vi "Configure Trace Buffer.vi"(4 "Trace Buffer Size (100000)":i32=100000, 6 "Trace Time Rule (1: Absolute)":i32(ring)=1 items=["Delta", "Absolute"], 7 "Trace Buffer Control (1: Never)":i32(ring)=1 items=["Next", "Never"], 8 "error in (no error)":errorcluster, 9 "Trace Buffer Data (2: SENS)":i32(ring)=2 items=["MATH", "LIM", "SENS"], 10 "Channel (0: Channel 1)":i32(ring) items=["Channel 1", "Channel 2"], 11 "VISA resource name":refnum<visa-resource-name>) -> (0 "error out":errorcluster, 3 "VISA resource name out":refnum<visa-resource-name>)   [LabVIEW 2020, in "Agilent B2900 Series.lvlib"]
doc: "Configures the settings for Trace Buffer. \n\n<B>Note:</B>\nCommand \":TRAC[c]:FEED LIM\" is not applicable for Agilent models B2961A, B2962A, B2961B, B2962B, B2961C and B2962C."
uses:
  Agilent B2900 Series.lvlib
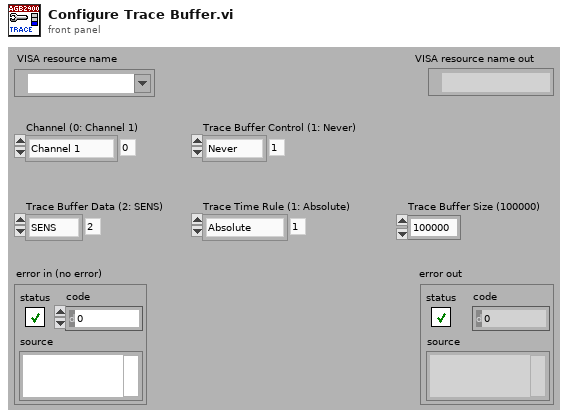
[diagram p1: front panel]
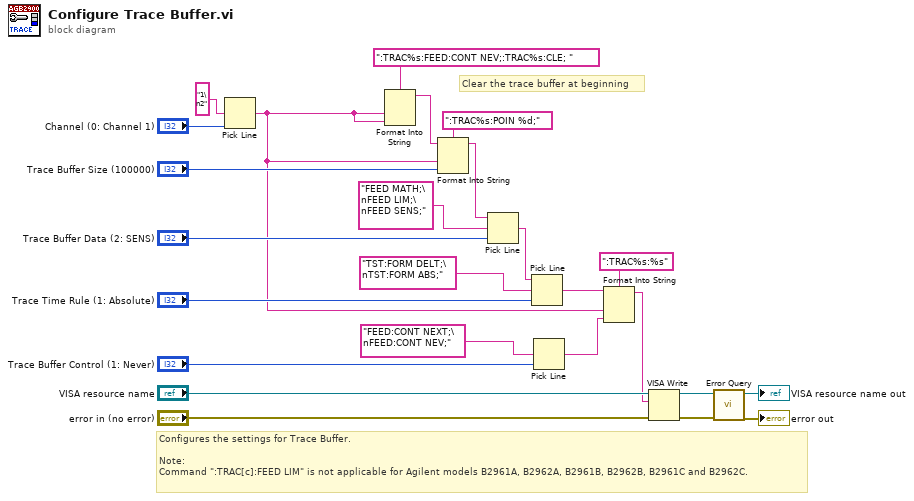
[diagram p0: block diagram]
diagram:
  # "Configures the settings for Trace Buffer. \n\nNote:\nCommand \":TRAC[c]:FEED LIM\" is not applicable for Agilent models B2961A, B2962A, B2961B, B2962B, B2961C and B2962C."
  # "Clear the trace buffer at beginning"
  n1 = Pick Line(multi-line string="1\n2" ("string (\"\")"), line index="Channel (0: Channel 1)") -> (output string=w4:string)  [unwired: 1 in]
  n2 = Format Into String(format string=":TRAC%s:FEED:CONT NEV;:TRAC%s:CLE; ", w4, w4) -> (resulting string=w8:string)  [unwired: 2 in, 1 out]
  n3 = Format Into String(format string=":TRAC%s:POIN %d;", initial string=w8, w4, "Trace Buffer Size (100000)") -> (resulting string=w7:string)  [unwired: 1 in, 1 out]
  n4 = Pick Line(string ("")=w7, multi-line string="FEED MATH;\nFEED LIM;\nFEED SENS;", line index="Trace Buffer Data (2: SENS)") -> (output string=w6:string)
  n5 = Pick Line(string ("")=w6, multi-line string="TST:FORM DELT;\nTST:FORM ABS;", line index="Trace Time Rule (1: Absolute)") -> (output string=w1:string)
  n6 = Pick Line(multi-line string="FEED:CONT NEXT;\nFEED:CONT NEV;", line index="Trace Buffer Control (1: Never)") -> (output string=w3:string)  [unwired: 1 in]
  n7 = Format Into String(format string=":TRAC%s:%s", initial string=w1, w4, w3) -> (resulting string=w2:string)  [unwired: 1 in, 1 out]
  n8 = VISA Write(VISA resource name="VISA resource name", write buffer=w2, error in (no error)="error in (no error)") -> (VISA resource name out=w15:refnum<visa-resource-name>, error out=w14:errorcluster)  [unwired: 1 out]
  n9 = call "Error Query.vi"("error in (no error)"=w14, "VISA resource name"=w15) -> ("error out"=→"error out":errorcluster, "VISA resource name out"=→"VISA resource name out":refnum<visa-resource-name>)  [unwired: 6 in, 2 out]
